vi "Insight_Create_Valid_Vector.vi"(8 "error in (no error)":errorcluster, 10 "Invalid Data Indices":i32[](array[numeric]), 11 "total data length":i32) -> (0 "error out":errorcluster, 2 "Valid Vector":i32[](array[numeric]))   [LabVIEW 2014]
doc: "Insight Photonic Solutions - v1.0\n\nThis VI creates a vector of indices (the \"Valid Vector\") for the Valid measurements in a sweep of the Insight laser, based on the Total Data Length and an array of Invalid Data Indices.\n\nUse this VI in combination with \"Insight_Reduce_Data_with_Valid-Vector\"."
panel:
  out "size(s) 2":i32
  out "size(s)":i32
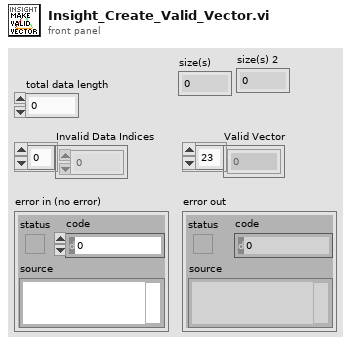
[diagram p1: front panel]
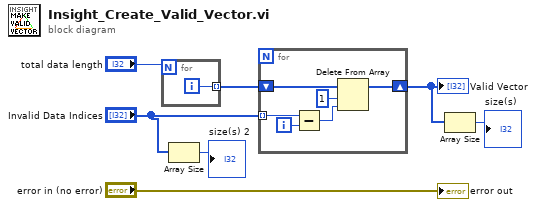
[diagram p0: block diagram]
diagram:
  n1 = for {
    N: "total data length" -> [_]
    tunnel: [w8] -> w7 mode=indexing
    i -> [w8]
  }
  n2 = Array Size(array="Invalid Data Indices") -> (size(s)=→"size(s) 2":i32)
  n3 = for {
    tunnel: "Invalid Data Indices" -> [w11] mode=indexing
    shift-right: [w13] -> w4
    shift-left: w7 -> [w14]
    i -> [w10]
    n4 = Subtract(x=w11, y=w10) -> (x-y=w9:i32)
    n5 = Delete From Array(array=w14, length=1, index=w9) -> (array with subset deleted=w13:i32[])  [unwired: 1 out]
  }
  "Valid Vector" <- w4
  n6 = Array Size(array=w4) -> (size(s)=→"size(s)":i32)
  "error out" <- "error in (no error)"
